vi "glb_complete.vi"() -> ()   [LabVIEW 2014]
panel:
  out "Complete":bool
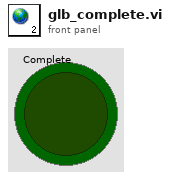
[diagram p1: front panel]
diagram:
